vi "QuVI_Wire (initial).vi"(2 "Stack in":refnum<class "QuSim.lvclass">[](array[class])) -> (8 "QuWire out":refnum<class "QuWire.lvclass">, 13 "Stack out":refnum<class "QuSim.lvclass">)   [LabVIEW 2020]
doc: "Initializes a qubit in the state |0> and provides a reference wire for circuit construction.\n\nThis VI serves as the fundamental starting point for any quantum circuit in the QuVI toolkit. It effectively initializes a single qubit in the ground state |0>.\n\nTo build a multi-qubit register, stack multiple instances of this VI vertically on the block diagram. The vertical connections aggregate the qubit count for the global state vector.\n\nTerminals:\n\n[Top] Stack in: Connect from the 'Stack out' of the previous qubit above. Leave unconnected for the first qubit (Qubit 0).\n\n[Bottom] Stack out: Connect to the 'Stack in' of the next qubit below.\n\n[Right] Quantum Wire Ref: The \"QuWire.\" Connect this to the left border of a Flat Sequence Structure."
uses:
  QuSim.lvclass
  QuWire/QuWire.lvclass
  C:/Users/HP/OneDrive/LabVIEW/Quantum Circuit Simulator/VIPM/QuVI 2020/QuSim/QuSim.lvclass
  SimAlg/PrllPerElement/PrllPerElmnt.lvclass
  SimAlg/QubitWise/QubitWiseMult.lvclass
  <vilib>/Utility/traverseref.llb/TRef TravTarget.ctl
  <vilib>/Utility/traverseref.llb/VI Scripting - Traverse.lvlib
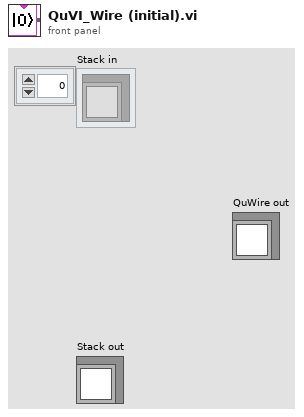
[diagram p1: front panel]
types:
  T1 = typedef "TRef TravTarget.ctl" = enum16{"FP", "BD", "Other"}
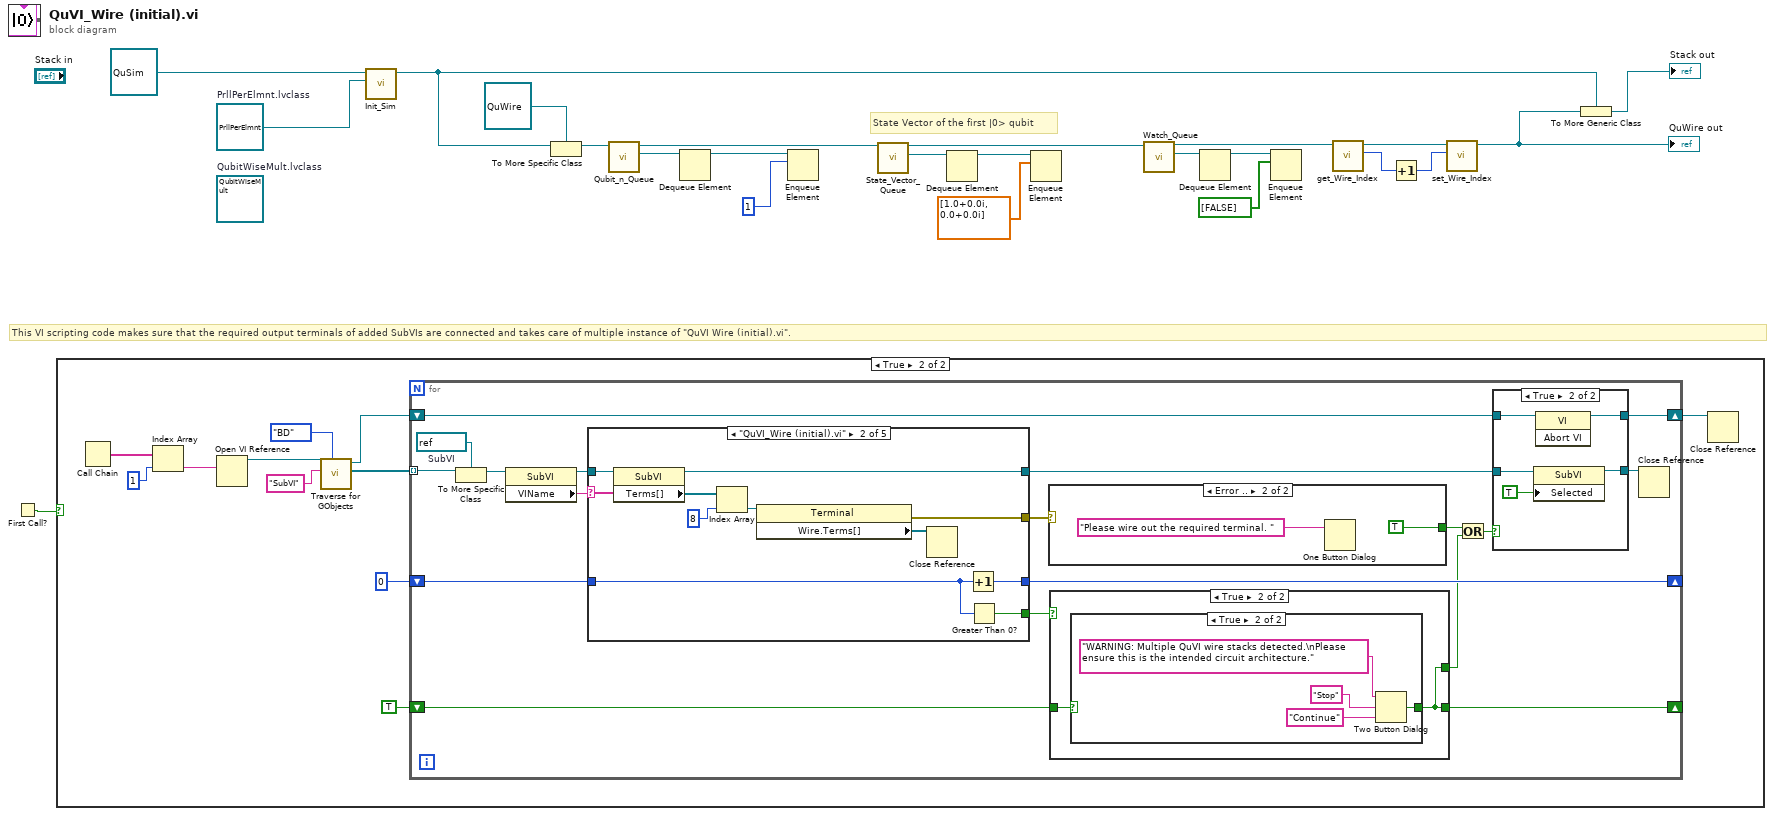
[diagram p0: block diagram]
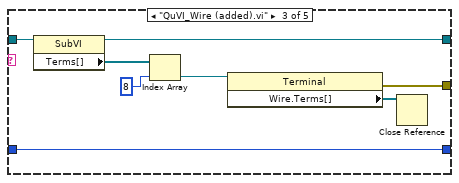
[diagram p4: hidden frame]
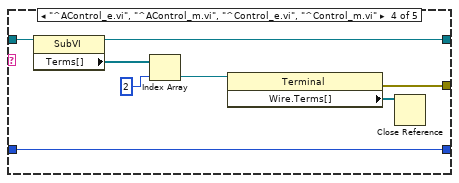
[diagram p5: hidden frame]
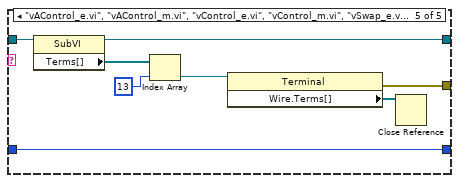
[diagram p6: hidden frame]
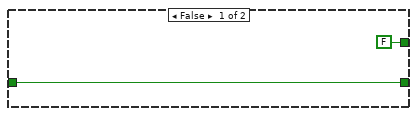
[diagram p8: hidden frame]
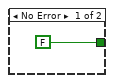
[diagram p10: hidden frame]
diagram:
  w5 = refnum<class "PrllPerElmnt.lvclass"> refnum  # PrllPerElmnt.lvclass
  (unwired) refnum<class "QubitWiseMult.lvclass"> refnum  # QubitWiseMult.lvclass
  # "This VI scripting code makes sure that the required output terminals of added SubVIs are connected and takes care of multiple instance of \"QuVI Wire (initial).vi\"."
  # "State Vector of the first |0> qubit"
  n1 = First Call?() -> (First Call?: T/F=w1:bool)
  n2 = case shown="True" w1 {
    frame False {
    }
    frame True {
      n3 = Call Chain() -> (call chain=w34:string[])
      n4 = Index Array(array=w34, index=1) -> (element=w32:string)
      n5 = Open VI Reference(vi path=w32) -> (vi reference=w31:refnum<vi>)  [unwired: 5 in, 1 out]
      n6 = call <vilib>:"Traverse for GObjects.vi"("Traverse Target"=TRef_TravTarget."BD", "Class Name"="SubVI", "VI Refnum"=w31) -> ("References"=w28:refnum<vi>[], "dup VI Refnum"=w27:refnum<vi>)  [unwired: 5 in, 2 out]
      n7 = for {
        tunnel: w28 -> [w52] mode=indexing
        shift-right: [w42] -> w26
        shift-left: w27 -> [w43]
        shift-right: [w45] -> _
        shift-left: 0 -> [w46]
        shift-right: [w36] -> _
        shift-left: TRUE -> [w37]
        w51 = refnum<vi> refnum  # SubVI
        n8 = To More Specific Class(target class=w51, reference=w52) -> (specific class reference=w50:refnum<vi>)  [unwired: 1 in, 1 out]
        n9 = property on="Property Node" class="SubVI"(reference=w50) -> (reference out=w48:refnum<vi>, "VIName"=w49:string)  [unwired: 1 in, 1 out]
        n10 = case shown="\"QuVI_Wire (initial).vi\"" w49 {
          tunnel: w48 -> [w54 w64 w72 w80 w88]
          tunnel: [_ w56 w68 w75 w83] -> w47
          tunnel: [w54 w60 w67 w74 w82] -> w40
          tunnel: w46 -> [w53 w57 w65 w73 w81]
          tunnel: [w53 w58 w65 w73 w81] -> w45
          tunnel: [_ w55 _ _ _] -> w44
          frame "False", Default {
          }
          frame "QuVI_Wire (initial).vi" {
            n11 = property on="Property Node" class="SubVI"(reference=w64) -> (reference out=w60:refnum<vi>, "Terms[]"=w63:refnum<vi>[])  [unwired: 1 in, 1 out]
            n12 = Index Array(array=w63, index=8) -> (element=w59:refnum<vi>)
            n13 = property on="Property Node" class="Terminal"(reference=w59) -> (error out=w56:errorcluster, "Wire.Terms[]"=w61:refnum<vi>[])  [unwired: 1 in, 1 out]
            n14 = Close Reference(reference=w61) -> ()  [unwired: 1 in, 1 out]
            n15 = Increment(x=w57) -> (x+1=w58:i32)
            n16 = Greater Than 0?(x=w57) -> (x > 0?=w55:bool)
          }
          frame "QuVI_Wire (added).vi" {
            n17 = property on="Property Node" class="SubVI"(reference=w72) -> (reference out=w67:refnum<vi>, "Terms[]"=w71:refnum<vi>[])  [unwired: 1 in, 1 out]
            n18 = Index Array(array=w71, index=8) -> (element=w66:refnum<vi>)
            n19 = property on="Property Node" class="Terminal"(reference=w66) -> (error out=w68:errorcluster, "Wire.Terms[]"=w69:refnum<vi>[])  [unwired: 1 in, 1 out]
            n20 = Close Reference(reference=w69) -> ()  [unwired: 1 in, 1 out]
          }
          frame "^AControl_e.vi", "^AControl_m.vi", "^Control_e.vi", "^Control_m.vi" {
            n21 = property on="Property Node" class="SubVI"(reference=w80) -> (reference out=w74:refnum<vi>, "Terms[]"=w79:refnum<vi>[])  [unwired: 1 in, 1 out]
            n22 = Index Array(array=w79, index=2) -> (element=w77:refnum<vi>)
            n23 = property on="Property Node" class="Terminal"(reference=w77) -> (error out=w75:errorcluster, "Wire.Terms[]"=w76:refnum<vi>[])  [unwired: 1 in, 1 out]
            n24 = Close Reference(reference=w76) -> ()  [unwired: 1 in, 1 out]
          }
          frame "vAControl_e.vi", "vAControl_m.vi", "vControl_e.vi", "vControl_m.vi", "vSwap_e.vi", "vSwap_m.vi" {
            n25 = property on="Property Node" class="SubVI"(reference=w88) -> (reference out=w82:refnum<vi>, "Terms[]"=w87:refnum<vi>[])  [unwired: 1 in, 1 out]
            n26 = Index Array(array=w87, index=13) -> (element=w85:refnum<vi>)
            n27 = property on="Property Node" class="Terminal"(reference=w85) -> (error out=w83:errorcluster, "Wire.Terms[]"=w84:refnum<vi>[])  [unwired: 1 in, 1 out]
            n28 = Close Reference(reference=w84) -> ()  [unwired: 1 in, 1 out]
          }
        }
        n29 = case shown="Error .." w47 {
          tunnel: [FALSE TRUE] -> w39
          frame No Error {
          }
          frame Error {
            n30 = One Button Dialog(message="Please wire out the required terminal. ") -> ()  [unwired: 1 in, 1 out]
          }
        }
        n31 = case shown="True" w44 {
          tunnel: w37 -> [w97 w99]
          tunnel: [w97 w98] -> w36
          tunnel: [FALSE ("T button?") w98] -> w35
          frame False {
          }
          frame True {
            n32 = case shown="True" w99 {
              selector: w99 -> [w100 _]
              tunnel: [w100 w102] -> w98
              frame False {
              }
              frame True {
                n33 = Two Button Dialog(message="WARNING: Multiple QuVI wire stacks detected.\nPlease ensure this is the intended circuit architecture.", 1:"Continue" ("F button name (\"Cancel\")"), 2:"Stop" ("T button name (\"OK\")")) -> (T button?=w102:bool)
              }
            }
          }
        }
        n34 = Or(x=w39, y=w35) -> (x .or. y?=w38:bool)
        n35 = case shown="True" w38 {
          tunnel: w43 -> [w90 w95]
          tunnel: [w90 w94] -> w42
          tunnel: [w89 w92] -> w41
          tunnel: w40 -> [w89 w91]
          frame False {
          }
          frame True {
            n36 = property on="Property Node" class="SubVI"(reference=w91, "Selected"=TRUE) -> (reference out=w92:refnum<vi>)  [unwired: 1 in, 1 out]
            n37 = invoke class="VI" method="Abort VI"(reference=w95) -> (reference out=w94:refnum<vi>)  [unwired: 2 in, 2 out]
          }
        }
        n38 = Close Reference(reference=w41) -> ()  [unwired: 1 in, 1 out]
      }
      n39 = Close Reference(reference=w26) -> ()  [unwired: 1 in, 1 out]
    }
  }
  n40 = call "Init_Sim.vi"("SimAlg.lvclass"=w5, "QuSim in"=refnum<class "QuSim.lvclass"> refnum ("QuSim.lvclass")) -> ("QuSim out"=w7:refnum<class "QuSim.lvclass">)  [unwired: 9 in]
  n41 = To More Specific Class(target class=refnum<class "QuWire.lvclass"> refnum ("Wire.lvclass"), reference=w7) -> (specific class reference=w20:refnum<class "QuWire.lvclass">)  [unwired: 1 in, 1 out]
  n42 = call "Qubit_n_Queue.vi"("QuWire in"=w20) -> ("Qubit n"=w21:refnum<queue>, "QuWire out"=w12:refnum<class "QuWire.lvclass">)  [unwired: 8 in, 1 out]
  n43 = Dequeue Element(queue=w21) -> (queue out=w22:refnum<queue>)  [unwired: 2 in, 3 out]
  n44 = Enqueue Element(queue=w22, element=1) -> ()  [unwired: 2 in, 3 out]
  n45 = call "State_Vector_Queue.vi"("QuWire in"=w12) -> ("State Vector Queue"=w13:refnum<queue>, "QuWire out"=w10:refnum<class "QuWire.lvclass">)  [unwired: 8 in, 1 out]
  n46 = Dequeue Element(queue=w13) -> (queue out=w14:refnum<queue>)  [unwired: 2 in, 3 out]
  n47 = Enqueue Element(queue=w14, element=cdb[] [1.0+0.0i, 0.0+0.0i]) -> ()  [unwired: 2 in, 3 out]
  n48 = call "Watch_Queue.vi"("QuWire in"=w10) -> ("Watch List"=w15:refnum<queue>, "QuWire out"=w11:refnum<class "QuWire.lvclass">)  [unwired: 8 in, 1 out]
  n49 = Dequeue Element(queue=w15) -> (queue out=w16:refnum<queue>)  [unwired: 2 in, 3 out]
  n50 = Enqueue Element(queue=w16, element=bool[] [FALSE]) -> ()  [unwired: 2 in, 3 out]
  n51 = call "get_Wire_Index.vi"("QuWire in"=w11) -> ("Wire Index"=w18:i32, "QuWire out"=w17:refnum<class "QuWire.lvclass">)  [unwired: 8 in, 1 out]
  n52 = Increment(x=w18) -> (x+1=w19:i32)
  n53 = call "set_Wire_Index.vi"("Wire Index"=w19, "QuWire in"=w17) -> ("QuWire out"=w9:refnum<class "QuWire.lvclass">)  [unwired: 8 in, 1 out]
  "QuWire out" <- w9
  n54 = To More Generic Class(target class=w7, reference=w9) -> (generic class reference=→"Stack out":refnum<class "QuSim.lvclass">)
